vi "test top level driver.vi"() -> ()   [LabVIEW 2016, in "labssh_thijs.lvlib"]
uses:
  labssh_thijs.lvlib
panel:
  in  "Input":string="whoami"
  out "prompt before $ sign":string
  out "output_new":string
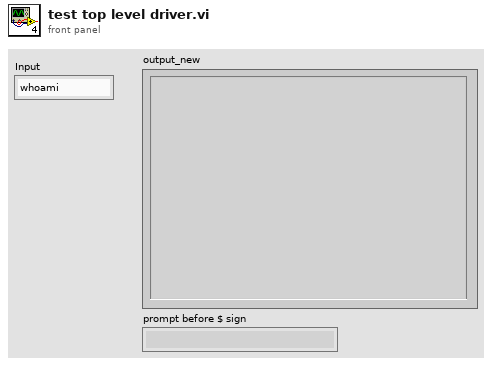
[diagram p1: front panel]
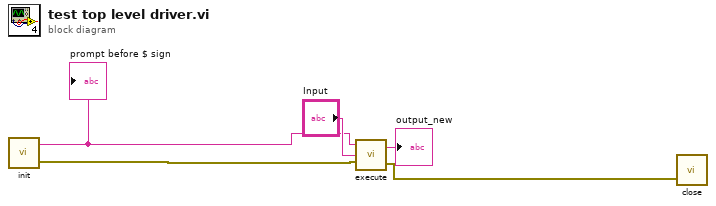
[diagram p0: block diagram]
diagram:
  n1 = call "init.vi"() -> ("error out"=w4:errorcluster, "prompt before $ sign"=w1:string)  [unwired: 2 in]
  "prompt before $ sign" <- w1
  n2 = call "execute.vi"("error in"=w4, "Input"="Input", "predetermined prompt without $"=w1) -> ("error out"=w2:errorcluster, "final match"=→"output_new":string)
  n3 = call "close.vi"("error in"=w2) -> ()  [unwired: 2 in, 1 out]
